vi "GlueCustomLinePattern.vi"(10 "Stereo Angle [mrad]":dbl=-26.0 format="%#_13g", 11 "Calibration Directory":path) -> ()   [LabVIEW 2016]
uses:
  <vilib>/LabVIEW Interface for Arduino/Type Defs/Arduino Resource.ctl
  <vilib>/LabVIEW Interface for Arduino/Type Defs/Board Type.ctl
  <vilib>/LabVIEW Interface for Arduino/Type Defs/Pin Mode.ctl
  <vilib>/Utility/file.llb/Read Delimited Spreadsheet (DBL).vi
  <vilib>/LabVIEW Interface for Arduino/LabVIEW Interface for Arduino.lvlib
panel:
  in  "Lines Control":enum32{"Repeated Lines", "Custom Lines"}(tab)
  in  "Relative Line Separations [mm]":dbl[][](array[numeric])=[[10.0, 0.0], [7.5, 5.0], [5.0, 5.0], [5.0, 5.0], [5.0, 5.0], [5.0, 12.5], [5.0, 5.0], [5.0, 5.0], [5.0, 5.0], [5.0, 5.0], [5.0, 5.0], [5.0, 5.0], [5.0, 5.0], [5.0, 5.0], [5.0, 5.0], [5.0, 5.0], [15.0, 5.0]] format="%#_13g"
  in  "Line Lengths [mm]":dbl[](array[numeric])=[60.0, 75.0, 75.0, 75.0, 75.0, 75.0, 75.0, 75.0, 75.0, 75.0, 75.0, 75.0, 75.0, 75.0, 75.0, 75.0, 37.5] format="%#_13g"
  in  "Line Speeds [mm/s]":dbl[][](array[numeric])=[[12.5, 12.5, 75.0, 75.0, 75.0, 75.0], [25.0, 25.0, 0.0, 0.0, 0.0, 0.0], [25.0, 25.0, 0.0, 0.0, 0.0, 0.0], [25.0, 25.0, 0.0, 0.0, 0.0, 0.0], [25.0, 25.0, 0.0, 0.0, 0.0, 0.0], [25.0, 25.0, 0.0, 0.0, 0.0, 0.0], [25.0, 25.0, 0.0, 0.0, 0.0, 0.0], [25.0, 25.0, 0.0, 0.0, 0.0, 0.0], [25.0, 25.0, 0.0, 0.0, 0.0, 0.0], [25.0, 25.0, 0.0, 0.0, 0.0, 0.0], [25.0, 25.0, 0.0, 0.0, 0.0, 0.0], [25.0, 25.0, 0.0, 0.0, 0.0, 0.0], [25.0, 25.0, 0.0, 0.0, 0.0, 0.0], [25.0, 25.0, 0.0, 0.0, 0.0, 0.0], [25.0, 25.0, 0.0, 0.0, 0.0, 0.0], [25.0, 25.0, 0.0, 0.0, 0.0, 0.0], [25.0, 25.0, 0.0, 0.0, 0.0, 0.0]] format="%#_13g"
  in  "AL - Left Start Relative to Corner [mm]":dbl[][](array[numeric])=[[62.5, 122.5], [-5.0, 35.0], [40.0, 35.0]]
  in  "AL - Line Lengths [mm]":dbl[](array[numeric])=[10.0, 35.0, 35.0]
  in  "AL - Line Speeds [mm/s]":dbl[][](array[numeric])=[[5.0, 5.0, 0.0], [12.5, 12.5, 0.0], [12.5, 12.5, 0.0]]
  in  "Outputs Tab":T1(tab)
  out "Running Positions (Repeated) [mm]":dbl[][](array[numeric])
  out "Running Positions (Custom) [mm]":dbl[][](array[numeric])
  out "All Positions [mm]":dbl[][](array[numeric])
  in  "Inputs Tab":T2(tab)
  out "Virtual Stave Map":path
  out "Stave Angle [rad]":dbl format="%#_13g"
  out "Total Angle [rad]":dbl
  in  "Module Number":i32=7
  in  "Glue Additional Lines":bool
  out "Arduino Resource":T3={"VISA resource"="GlueCTRL", "Board Type"=enum."Uno", "Connection Type"=enum."USB / Serial", "Bytes Per Packet (15)"=15}
  in  "Digital I/O Pin":u8=7
  in  "Default Axis Speeds":T5={"X [mm/s]"=25.0, "Y [mm/s]"=25.0, "Z [mm/s]"=25.0}
  in  "Pause After Gluing [ms]":dbl=250.0 format="%#_13g"
  out "N Lines (Repeated)":i32
  out "N Lines (Custom)":i32
  in  "Fine Axis Speeds":T5={"X [mm/s]"=25.0, "Y [mm/s]"=25.0, "Z [mm/s]"=25.0}
  in  "Dry Run":bool
  in  "Positions [mm]":dbl[][](array[numeric])
  in  "OK Button":bool
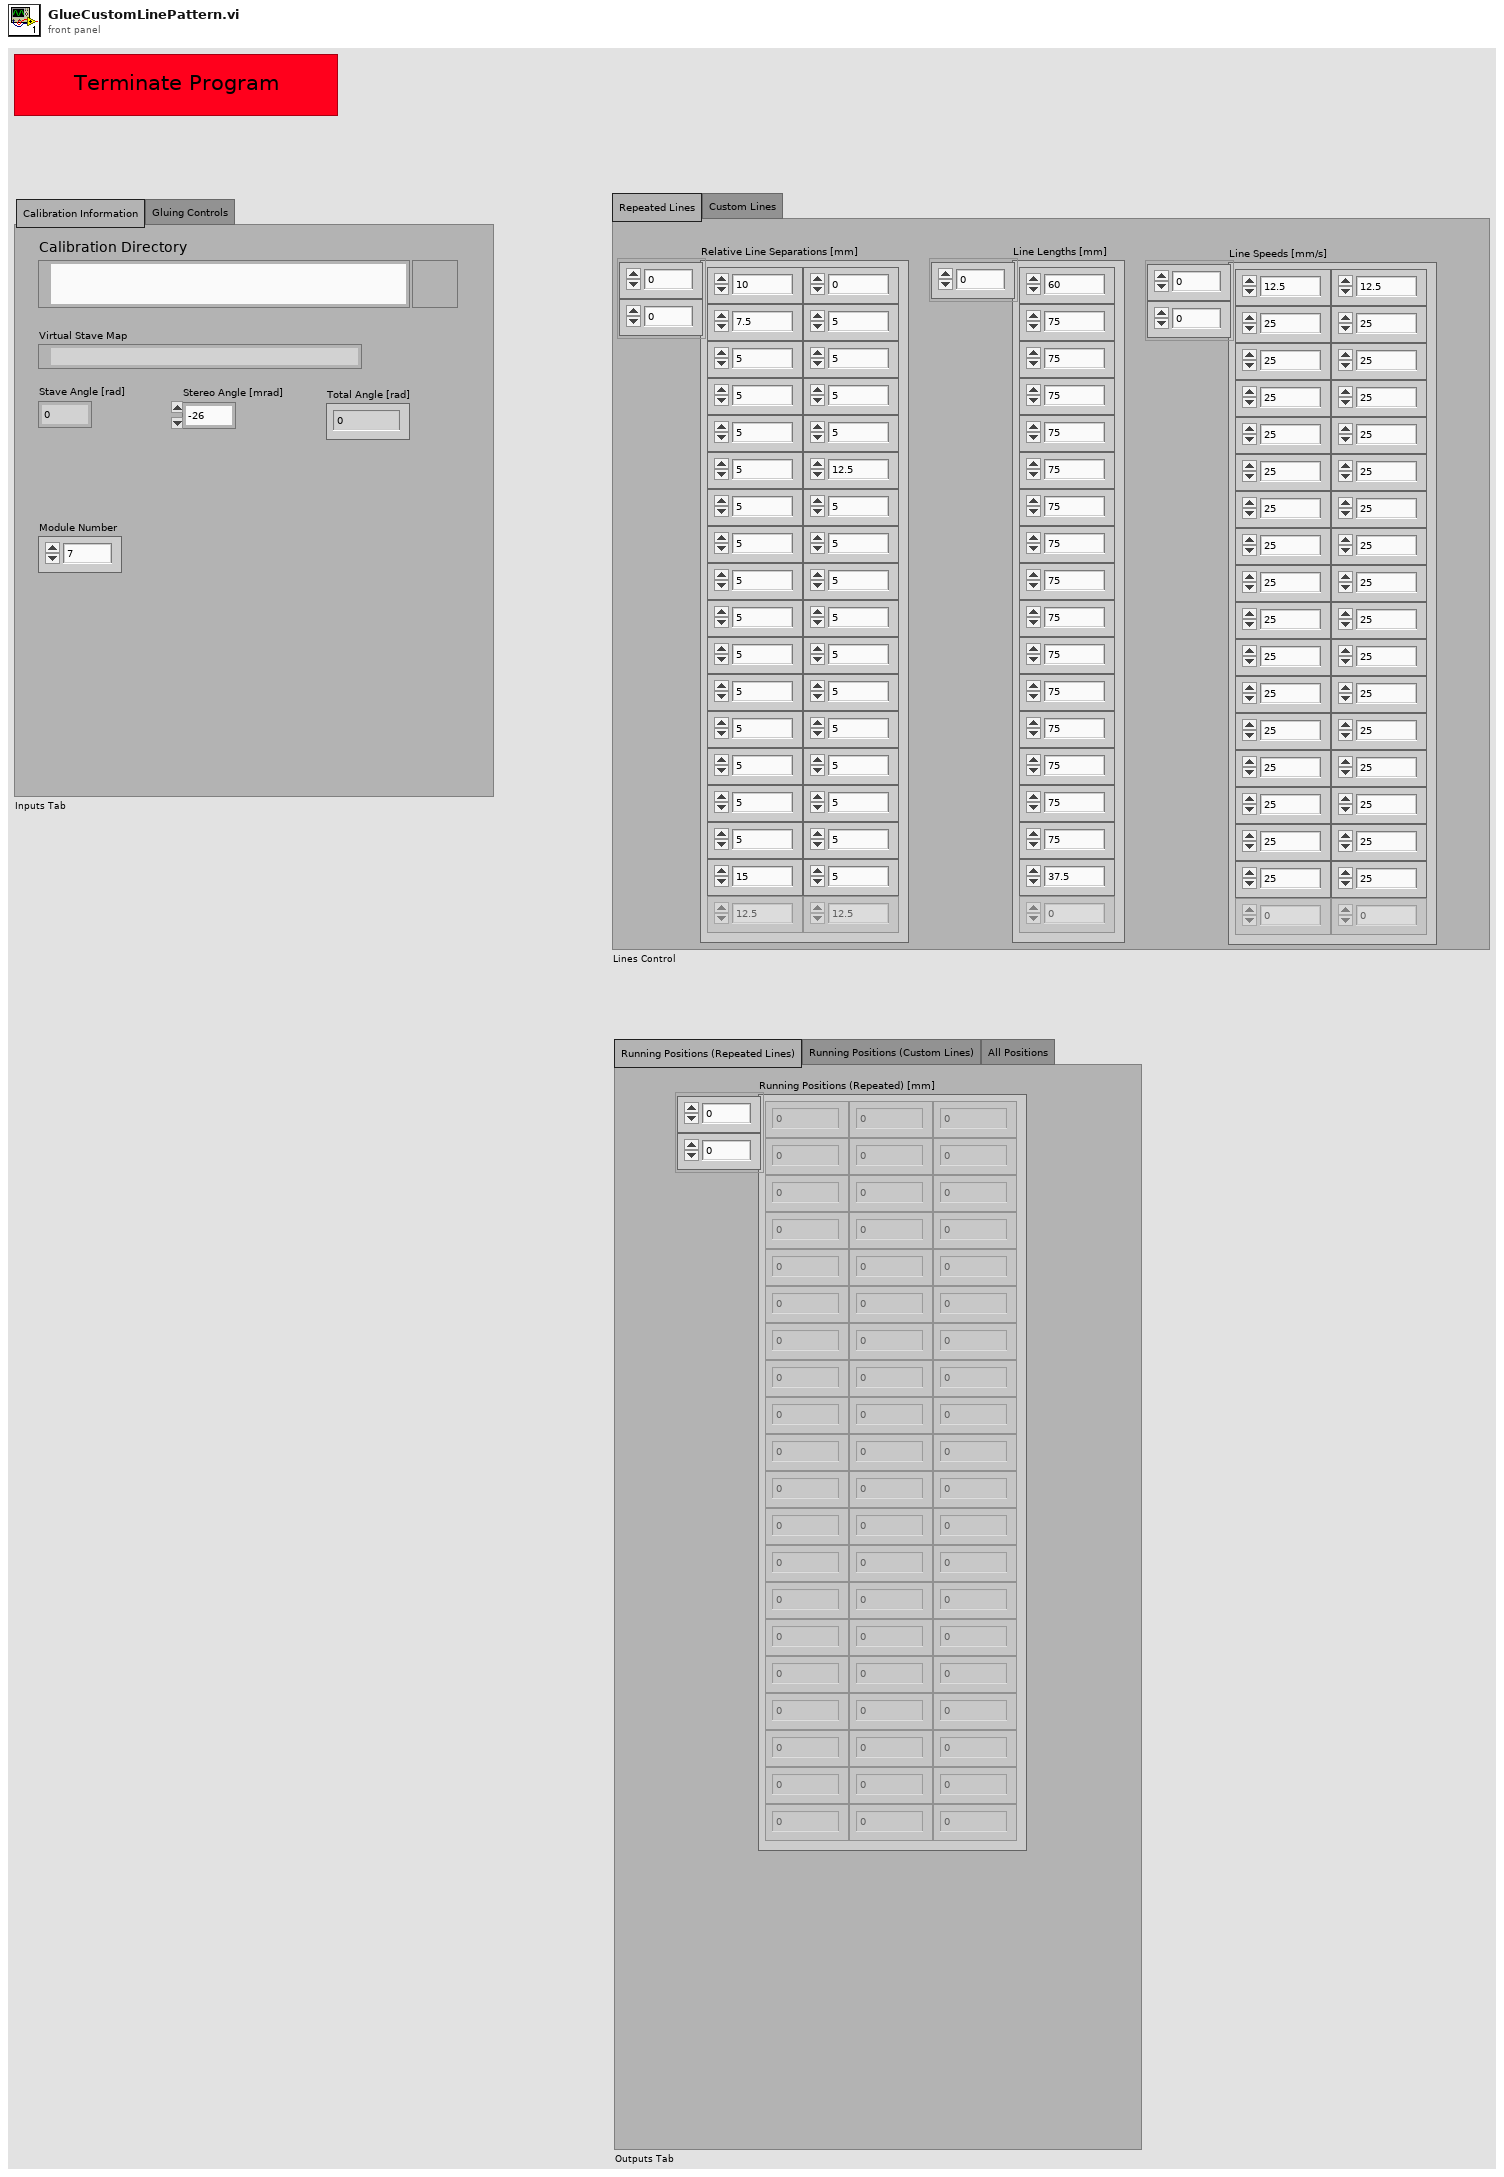
[diagram p1: front panel]
types:
  T1 = enum32{"Running Positions (Repeated Lines)", "Running Positions (Custom Lines)", "All Positions"}
  T2 = enum32{"Calibration Information", "Gluing Controls"}
  T3 = typedef "LabVIEW Interface for Arduino.lvlib/Arduino Resource.ctl" = cluster{"VISA resource":refnum<visa-resource-name>, "Board Type":T4, "Connection Type":enum8{"USB / Serial"}, "Bytes Per Packet (15)":u8}
  T4 = typedef "LabVIEW Interface for Arduino.lvlib/Board Type.ctl" = enum16{"Uno", "Dimuelanove w/Atmega 328", "Mega 2560"}
  T5 = cluster{"X [mm/s]":dbl, "Y [mm/s]":dbl, "Z [mm/s]":dbl}
  T6 = typedef "LabVIEW Interface for Arduino.lvlib/Pin Mode.ctl" = enum8{"Input", "Output"}
  T7 = cluster{"Final X":dbl, "Final Y":dbl, "Final Z":dbl}
  T8 = cluster{"Line Separation [mm]":dbl, "Line Separation [mm]":dbl, "Z [mm/s]":dbl}
  T9 = cluster{"Numeric Control":dbl, "Numeric Control":dbl, "Z [mm/s]":dbl}
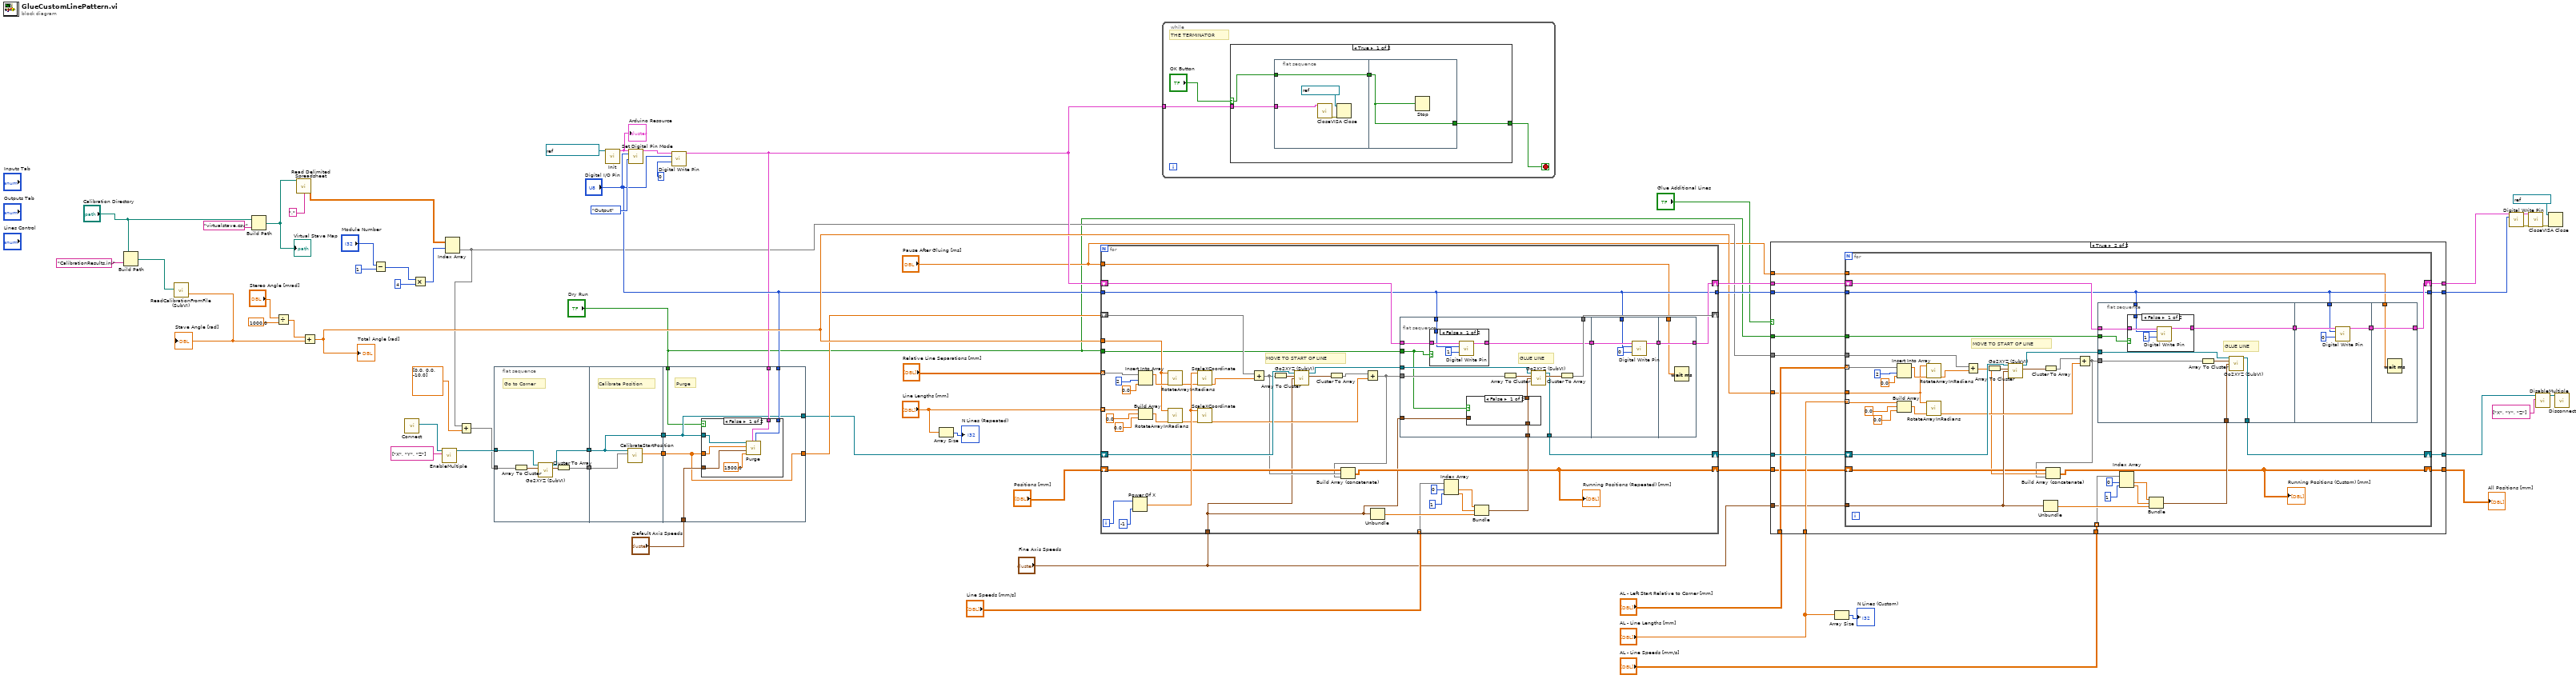
[diagram p0: block diagram]
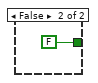
[diagram p7: hidden frame]
diagram:
  n1 = Build Path(base path="Calibration Directory", name or relative path="CalibrationResults.ini") -> (appended path=w58:path)
  n2 = call "ReadCalibrationFromFile (SubVI).vi"("Calibration file path"=w58) -> ("Angle"=w55:dbl)  [unwired: 12 in, 6 out]
  "Stave Angle [rad]" <- w55
  n3 = Build Path(base path="Calibration Directory", name or relative path="virtualstave.csv") -> (appended path=w63:path)
  "Virtual Stave Map" <- w63
  n4 = Divide(x="Stereo Angle [mrad]", y=1000.0) -> (x/y=w54:dbl)
  n5 = call-poly <vilib>:"Read Delimited Spreadsheet.vi"("file path (dialog if empty)"=w63, "delimiter (\\t)"="," ("delimiter (\\t)")) -> ("all rows"=w59:dbl[][])  [unwired: 8 in, 5 out]
  n6 = Add(x=w54, y=w55) -> (x+y=w18:dbl)
  "Total Angle [rad]" <- w18
  n7 = Subtract(x="Module Number", y=1) -> (x-y=w60:i32)
  n8 = call "Connect.vi"() -> ("controller"=w50:refnum<k24>)  [unwired: 10 in, 1 out]
  n9 = Multiply(x=w60, y=4) -> (x*y=w61:i32)
  n10 = call "EnableMultiple.vi"("axis names"=string[] ["X", "Y", "Z"] ("Axes Names"), "controller in"=w50) -> ("controller out"=w17:refnum<k24>)  [unwired: 8 in, 1 out]
  n11 = Index Array(array=w59, index (row)=w61) -> (element=w7:dbl[])  [unwired: 1 in]
  n12 = Add(x=w7, y=dbl[] [0.0, 0.0, -10.0]) -> (x+y=w5:dbl[])
  n13 = flat-sequence {
    tunnel: w17 -> [w68]
    tunnel: [w67] -> w16
    tunnel: w5 -> [w66]
    tunnel: [w65] -> w15
    tunnel: w16 -> [w72]
    tunnel: w15 -> [w73]
    tunnel: [w72] -> w14
    tunnel: [w71] -> w13
    tunnel: w14 -> [w76]
    tunnel: w13 -> [w74]
    tunnel: [w74] -> w12
    tunnel: "Default Axis Speeds" -> [w79]
    tunnel: "Digital I/O Pin" -> [w78]
    tunnel: w9 -> [w77]
    tunnel: [w76] -> w8
    tunnel: "Dry Run" -> [w75]
    frame #0 {
      # "Go to Corner"
      n14 = Array To Cluster(array=w66) -> (cluster=w70:cluster{"[0]":dbl, "[1]":dbl, "[2]":dbl})
      n15 = call "Go2XYZ (SubVI).vi"(".NET Refnum in"=w68, "Go to Coordinates"=w70) -> (".NET Refnum out"=w67:refnum<k24>, "Final Position"=w69:T7)  [unwired: 9 in, 3 out]
      n16 = Cluster To Array(cluster=w69) -> (array=w65:dbl[])
    }
    frame #1 {
      # "Calibrate Position"
      n17 = call "CalibrateStartPosition.vi"("Start Position [mm]"=w73, ".NET Refnum In"=w72) -> ("Final Position [mm]"=w71:dbl[])  [unwired: 9 in]
    }
    frame #2 {
      # "Purge"
      n18 = case shown="False" w75 {
        tunnel: w79 -> [w82 _]
        tunnel: w78 -> [w85 _]
        tunnel: w77 -> [w84 _]
        tunnel: w76 -> [w80 _]
        tunnel: w74 -> [w81 _]
        frame False {
          n19 = call "Purge.vi"("Digital I/O Pin"=w85, "Arduino Resource"=w84, "Purge Time [ms]"=1500.0, "Axis Speeds"=w82, "Start Position [mm]"=w81, ".NET Refnum In"=w80) -> ()  [unwired: 6 in]
        }
        frame True {
        }
      }
    }
  }
  n20 = call <vilib>:"Init.vi"("VISA resource"=refnum<visa-resource-name> "GlueCTRL") -> ("Arduino Resource"=w44:T3)  [unwired: 17 in, 1 out]
  "Arduino Resource" <- w44
  n21 = call <vilib>:"Set Digital Pin Mode.vi"("Arduino Resource"=w44, "Digital I/O Pin"="Digital I/O Pin", "Pin Mode (Input)"=Pin_Mode."Output") -> ("Arduino Resource"=w47:T3)  [unwired: 11 in, 1 out]
  n22 = call <vilib>:"Digital Write Pin.vi"("Arduino Resource"=w47, "Digital I/O Pin (0)"="Digital I/O Pin", "Value (0)"=u8 0) -> ("Arduino Resource"=w9:T3)  [unwired: 11 in, 1 out]
  n23 = Array Size(array="Line Lengths [mm]") -> (size(s)=→"N Lines (Repeated)":i32)
  n24 = for {
    tunnel: "Relative Line Separations [mm]" -> [w124] mode=indexing
    tunnel: "Line Lengths [mm]" -> [w125] mode=indexing
    tunnel: w18 -> [w119]
    shift-right: [w110] -> _
    shift-left: w12 -> [w114]
    tunnel: "Line Speeds [mm/s]" -> [w107] mode=indexing
    shift-right: [w102] -> w29
    shift-left: w8 -> [w101]
    shift-right: [w97] -> w27
    shift-left: w9 -> [w99]
    shift-right: [w90] -> w22
    shift-left: "Positions [mm]" -> [w94]
    tunnel: "Digital I/O Pin" -> [w96]
    tunnel: [w96] -> w25
    tunnel: "Pause After Gluing [ms]" -> [w88]
    tunnel: "Fine Axis Speeds" -> [w87]
    tunnel: "Dry Run" -> [w86]
    i -> [w93]
    # "MOVE TO START OF LINE"
    n25 = Power Of X(1:-1 ("x"), 2:w93) -> (0:w117:dbl)
    n26 = Insert Into Array(array=w124, index=2, new element=0.0 ("new element/subarray")) -> (w121:dbl[])
    n27 = Build Array(w125, 0.0 ("element"), 0.0 ("element")) -> (w120:dbl[])
    n28 = call "RotateArrayInRadians.vi"("X,Y,Z Input"=w121, "Angle"=w119) -> ("X,Y,Z Output"=w115:dbl[])  [unwired: 9 in]
    n29 = call "RotateArrayInRadians.vi"("X,Y,Z Input"=w120, "Angle"=w119) -> ("X,Y,Z Output"=w116:dbl[])  [unwired: 9 in]
    n30 = call "ScaleXCoordinate.vi"("X, Y, Z Input"=w115, "Scale"=w117) -> ("-X, Y, Z Output"=w112:dbl[])  [unwired: 9 in]
    n31 = call "ScaleXCoordinate.vi"("X, Y, Z Input"=w116, "Scale"=w117) -> ("-X, Y, Z Output"=w95:dbl[])  [unwired: 9 in]
    n32 = Add(x=w114, y=w112) -> (x+y=w92:dbl[])
    n33 = Array To Cluster(array=w92) -> (cluster=w113:cluster{"[0]":dbl, "[1]":dbl, "[2]":dbl})
    n34 = call "Go2XYZ (SubVI).vi"(".NET Refnum in"=w101, "Go to Coordinates"=w113, "Axis Speeds"=w87) -> (".NET Refnum out"=w111:refnum<k24>, "Final Position"=w118:T7)  [unwired: 8 in, 3 out]
    n35 = Cluster To Array(cluster=w118) -> (array=w100:dbl[])
    n36 = Add(x=w100, y=w95) -> (x+y=w91:dbl[])
    n37 = Build Array (concatenate)(w94, w92, w91) -> (w90:dbl[][])
    "Running Positions (Repeated) [mm]" <- w90
    n38 = Unbundle(w87) -> ("Z [mm/s]"=w109:dbl)  [unwired: 2 out]
    n39 = flat-sequence {
      tunnel: [w137] -> w110
      tunnel: w108 -> [w129]
      tunnel: [w136] -> w102
      tunnel: [w135] -> w98
      tunnel: w96 -> [w133]
      tunnel: w99 -> [w134]
      tunnel: w111 -> [w138]
      tunnel: w91 -> [w140]
      tunnel: w87 -> [w131]
      tunnel: w86 -> [w132]
      tunnel: w98 -> [w152]
      tunnel: w96 -> [w150]
      tunnel: [w151] -> w89
      tunnel: [w154] -> w97
      tunnel: w89 -> [w154]
      tunnel: w88 -> [w153]
      frame #0 {
        # "GLUE LINE"
        n40 = case shown="False" w132 {
          tunnel: [w147 w148] -> w135
          tunnel: w134 -> [w146 w148]
          tunnel: w133 -> [w145 _]
          frame False {
            n41 = call <vilib>:"Digital Write Pin.vi"("Arduino Resource"=w146, "Digital I/O Pin (0)"=w145, "Value (0)"=u8 1) -> ("Arduino Resource"=w147:T3)  [unwired: 11 in, 1 out]
          }
          frame True {
          }
        }
        n42 = case shown="False" w132 {
          tunnel: w131 -> [_ w143]
          tunnel: [w142 w143] -> w130
          tunnel: w129 -> [w142 _]
          frame False {
          }
          frame True {
          }
        }
        n43 = Array To Cluster(array=w140) -> (cluster=w139:cluster{"[0]":dbl, "[1]":dbl, "[2]":dbl})
        n44 = call "Go2XYZ (SubVI).vi"(".NET Refnum in"=w138, "Go to Coordinates"=w139, "Axis Speeds"=w130) -> (".NET Refnum out"=w136:refnum<k24>, "Final Position"=w141:T7)  [unwired: 8 in, 3 out]
        n45 = Cluster To Array(cluster=w141) -> (array=w137:dbl[])
      }
      frame #1 {
        n46 = call <vilib>:"Digital Write Pin.vi"("Arduino Resource"=w152, "Digital I/O Pin (0)"=w150, "Value (0)"=u8 0) -> ("Arduino Resource"=w151:T3)  [unwired: 11 in, 1 out]
      }
      frame #2 {
        n47 = Wait (ms)(milliseconds to wait=w153) -> ()  [unwired: 1 out]
      }
    }
    n48 = Index Array(array=w107, index #1=0 ("index"), index #2=1 ("index")) -> (element #1=w103:dbl, element #2=w104:dbl)
    n49 = Bundle("Line Separation [mm]"=w103, "Line Separation [mm]"=w104, "Z [mm/s]"=w109) -> (w108:T8)  [unwired: 1 in]
  }
  n50 = while {
    tunnel: w9 -> [w156]
    stop <- w155 stop-if-true
    # "THE TERMINATOR"
    n51 = case shown="True" "OK Button" {
      selector: "OK Button" -> [w161 _]
      tunnel: w156 -> [w159 _]
      tunnel: [w158 FALSE] -> w155
      frame True {
        n52 = flat-sequence {
          tunnel: w161 -> [w163]
          tunnel: [w163] -> w160
          tunnel: w159 -> [w162]
          tunnel: w160 -> [w166]
          tunnel: [w166] -> w158
          frame #0 {
            n53 = call <vilib>:"Close.vi"("Arduino Resource"=w162) -> ("error out"=w164:errorcluster)  [unwired: 14 in]
            n54 = VISA Close(VISA resource name=refnum<visa-resource-name> "GlueCTRL", error in (no error)=w164) -> ()  [unwired: 1 out]
          }
          frame #1 {
            n55 = Stop(stop? (T)=w166) -> ()
          }
        }
      }
      frame False {
      }
    }
  }
  n56 = case shown="True" "Glue Additional Lines" {
    tunnel: "AL - Left Start Relative to Corner [mm]" -> [_ w182]
    tunnel: "AL - Line Lengths [mm]" -> [_ w181]
    tunnel: "AL - Line Speeds [mm/s]" -> [_ w180]
    tunnel: w29 -> [w171 w187]
    tunnel: [w171 w186] -> w28
    tunnel: w27 -> [w170 w185]
    tunnel: [w170 w184] -> w26
    tunnel: w25 -> [w169 w183]
    tunnel: [w169 w179] -> w24
    tunnel: w18 -> [_ w178]
    tunnel: w7 -> [_ w176]
    tunnel: "Fine Axis Speeds" -> [_ w177]
    tunnel: w22 -> [w168 w175]
    tunnel: [w168 w174] -> w21
    tunnel: "Pause After Gluing [ms]" -> [_ w173]
    tunnel: "Dry Run" -> [_ w172]
    frame False {
    }
    frame True {
      n57 = for {
        shift-right: [w208] -> w186
        shift-left: w187 -> [w211]
        shift-right: [w206] -> w184
        shift-left: w185 -> [w207]
        tunnel: w182 -> [w218] mode=indexing
        tunnel: w181 -> [w217] mode=indexing
        tunnel: w180 -> [w197] mode=indexing
        tunnel: w178 -> [w216]
        tunnel: w177 -> [w198]
        tunnel: w176 -> [w195]
        shift-right: [w192] -> w174
        shift-left: w175 -> [w194]
        tunnel: w183 -> [w204]
        tunnel: [w204] -> w179
        tunnel: w173 -> [w189]
        tunnel: w172 -> [w188]
        # "MOVE TO START OF LINE"
        n58 = Insert Into Array(array=w218, index=2, new element=0.0 ("new element/subarray")) -> (w220:dbl[])
        n59 = Build Array(w217, 0.0 ("element"), 0.0 ("element")) -> (w219:dbl[])
        n60 = call "RotateArrayInRadians.vi"("X,Y,Z Input"=w220, "Angle"=w216) -> ("X,Y,Z Output"=w212:dbl[])  [unwired: 9 in]
        n61 = call "RotateArrayInRadians.vi"("X,Y,Z Input"=w219, "Angle"=w216) -> ("X,Y,Z Output"=w210:dbl[])  [unwired: 9 in]
        n62 = Add(x=w195, y=w212) -> (x+y=w193:dbl[])
        n63 = Array To Cluster(array=w193) -> (cluster=w214:cluster{"[0]":dbl, "[1]":dbl, "[2]":dbl})
        n64 = call "Go2XYZ (SubVI).vi"(".NET Refnum in"=w211, "Go to Coordinates"=w214, "Axis Speeds"=w198) -> (".NET Refnum out"=w205:refnum<k24>, "Final Position"=w215:T7)  [unwired: 8 in, 3 out]
        n65 = Unbundle(w198) -> ("Z [mm/s]"=w203:dbl)  [unwired: 2 out]
        n66 = Cluster To Array(cluster=w215) -> (array=w213:dbl[])
        n67 = Add(x=w213, y=w210) -> (x+y=w191:dbl[])
        n68 = Build Array (concatenate)(w194, w193, w191) -> (w192:dbl[][])
        "Running Positions (Custom) [mm]" <- w192
        n69 = flat-sequence {
          tunnel: [w233] -> w209
          tunnel: [w232] -> w208
          tunnel: w207 -> [w231]
          tunnel: w205 -> [w230]
          tunnel: w191 -> [w229]
          tunnel: w204 -> [w227]
          tunnel: w196 -> [w226]
          tunnel: w188 -> [w225]
          tunnel: w209 -> [w242]
          tunnel: w204 -> [w239]
          tunnel: [w241] -> w190
          tunnel: [w244] -> w206
          tunnel: w190 -> [w244]
          tunnel: w189 -> [w243]
          frame #0 {
            # "GLUE LINE"
            n70 = case shown="False" w225 {
              tunnel: [w237 w238] -> w233
              tunnel: w231 -> [w235 w238]
              tunnel: w227 -> [w234 _]
              frame False {
                n71 = call <vilib>:"Digital Write Pin.vi"("Arduino Resource"=w235, "Digital I/O Pin (0)"=w234, "Value (0)"=u8 1) -> ("Arduino Resource"=w237:T3)  [unwired: 11 in, 1 out]
              }
              frame True {
              }
            }
            n72 = Array To Cluster(array=w229) -> (cluster=w228:cluster{"[0]":dbl, "[1]":dbl, "[2]":dbl})
            n73 = call "Go2XYZ (SubVI).vi"(".NET Refnum in"=w230, "Go to Coordinates"=w228, "Axis Speeds"=w226) -> (".NET Refnum out"=w232:refnum<k24>)  [unwired: 8 in, 4 out]
          }
          frame #1 {
            n74 = call <vilib>:"Digital Write Pin.vi"("Arduino Resource"=w242, "Digital I/O Pin (0)"=w239, "Value (0)"=u8 0) -> ("Arduino Resource"=w241:T3)  [unwired: 11 in, 1 out]
          }
          frame #2 {
            n75 = Wait (ms)(milliseconds to wait=w243) -> ()  [unwired: 1 out]
          }
        }
        n76 = Index Array(array=w197, index #1=0 ("index"), index #2=1 ("index")) -> (element #1=w199:dbl, element #2=w200:dbl)
        n77 = Bundle("Numeric Control"=w199, "Numeric Control"=w200, "Z [mm/s]"=w203) -> (w196:T9)  [unwired: 1 in]
      }
    }
  }
  "All Positions [mm]" <- w21
  n78 = Array Size(array="AL - Line Lengths [mm]") -> (size(s)=→"N Lines (Custom)":i32)
  n79 = call <vilib>:"Digital Write Pin.vi"("Arduino Resource"=w26, "Digital I/O Pin (0)"=w24) -> ("Arduino Resource"=w42:T3, "error out"=w41:errorcluster)  [unwired: 12 in]
  n80 = call <vilib>:"Close.vi"("Arduino Resource"=w42, "error in"=w41) -> ("error out"=w40:errorcluster)  [unwired: 13 in]
  n81 = call "DisableMultiple.vi"("axis names"=string[] ["X", "Y", "Z"], "controller in"=w28) -> ("controller out"=w39:refnum<k24>)  [unwired: 8 in, 1 out]
  n82 = VISA Close(VISA resource name=refnum<visa-resource-name> "GlueCTRL", error in (no error)=w40) -> ()  [unwired: 1 out]
  n83 = call "Disconnect.vi"("controller"=w39) -> ()  [unwired: 10 in, 1 out]
